vi "Handle Error.vi"(8 "error in (no error)":errorcluster, 11 "Proxy in":refnum<class "Proxy.lvclass">) -> (0 "error out":errorcluster, 2 "stop actor?":bool=TRUE, 3 "Proxy out":refnum<class "Proxy.lvclass">)   [LabVIEW 2014]
doc: "(<B>Filename</B>: Actor Framework.lvlib:Actor.lvclass:Handle Error.vi)\n\nDefines how the actor handles an error that occurred while processing a message. By default, this method does nothing except stop the actor."
uses:
  Proxy.lvclass
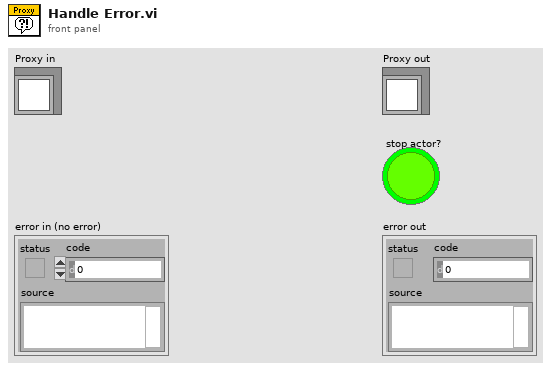
[diagram p1: front panel]
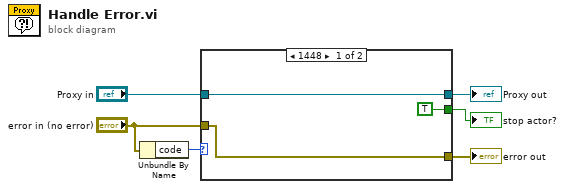
[diagram p0: block diagram]
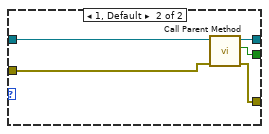
[diagram p2: hidden frame]
diagram:
  n1 = Unbundle By Name("error in (no error)") -> ("code"=w1:i32)
  n2 = case shown="1448" w1 {
    tunnel: [w7 w14] -> w6
    tunnel: [TRUE ("status") w13] -> w5
    tunnel: [w8 w12] -> w4
    tunnel: "error in (no error)" -> [w7 w11]
    tunnel: "Proxy in" -> [w8 w10]
    frame 1448 {
    }
    frame 1, Default {
      n3 = call-parent "Call Parent Method"("error in (no error)"=w11, "Actor in"=w10) -> ("error out"=w14:errorcluster, "stop actor?"=w13:bool, "Actor out"=w12:refnum<class "Proxy.lvclass">)  [unwired: 7 in]
    }
  }
  "Proxy out" <- w4
  "error out" <- w6
  "stop actor?" <- w5
